vi "Autonomous Independent.vi"() -> ()   [LabVIEW 2011]
doc: "This VI is called when autonomous begins, and will automatically be terminated when autonomous ends. You can carry out timed or sensor driven robot movement independently without needing to return to the caller."
uses:
  <vilib>/Rock Robotics/WPI/Relay/WPI_RelayValue.ctl
  Robot Global Data.vi
panel:
  in  "Recording Auton":bool
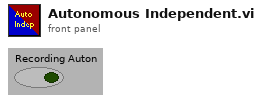
[diagram p1: front panel]
types:
  T1 = typedef "WPI_MotorControlDeviceRef.ctl" = cluster{"DeviceStatus":errorcluster, "Type":enum16{"PWM", "CAN"}, "PWM":cluster{"Digital Module":T2, "PWM Channel":T3, "DeadBand":T4}, "CAN":cluster{"Device Number":u8, "Control Mode":T5, "Semaphore":T6, "Max Vout":dbl}, "Invert":bool, "TransformRef":T7, "InvTransformRef":T7}
  T2 = typedef "FPGA_TypedefDigitalModule.ctl" = enum16{"Digital Module 1", "Digital Module 2"}
  T3 = typedef "FPGA_DIOPWMChannel.ctl" = enum8{"PWM 1", "PWM 2", "PWM 3", "PWM 4", "PWM 5", "PWM 6", "PWM 7", "PWM 8", "PWM 9", "PWM 10", "Invalid"}
  T4 = typedef "WPI_PWMDeadband.ctl" = cluster{"Name":string, "maxPositivePwm":i32, "minPositivePwm":i32, "centerPwm":i32, "maxNegativePwm":i32, "minNegativePwm":i32, "angularRange":u16}
  T5 = typedef "WPI_CANJaguar_ControlMode.ctl" = enum8{"Percent VBus", "Current", "Speed", "Position", "Voltage"}
  T6 = typedef "Semaphore RefNum" = refnum<k1>
  T7 = typedef "WPI_PWMTransform_ConPane.ctl" = refnum<vi>
  T8 = typedef "WPI_ServoDeviceRef.ctl" = cluster{"DeviceStatus":errorcluster, "Digital Module":T2, "PWM Channel":T3, "DeadBand":T4}
  T9 = typedef "WPI_RelayValue.ctl" = enum16{"Off", "On", "Forward", "Reverse"}
  T10 = typedef "WPI_RelayDevRef.ctl" = cluster{"DevStatus":errorcluster, "Relay Channel":T11, "Digital Module":T2, "Relay Direction":T12}
  T11 = typedef "FPGA_DIORelayChannel.ctl" = enum8{"Relay 1", "Relay 2", "Relay 3", "Relay 4", "Relay 5", "Relay 6", "Relay 7", "Relay 8", "Invalid"}
  T12 = typedef "WPI_RelayDirection.ctl" = enum16{"Both directions", "Forward only", "Reverse only"}
  T13 = typedef "WPI_DigitalInputDevRef.ctl" = cluster{"DevStatus":errorcluster, "DIO Channel":T14, "Digital Module":T2}
  T14 = typedef "FPGA_DIOChannel.ctl" = enum8{"DIO 1", "DIO 2", "DIO 3", "DIO 4", "DIO 5", "DIO 6", "DIO 7", "DIO 8", "DIO 9", "DIO 10", "DIO 11", "DIO 12", "DIO 13", "DIO 14", "Invalid"}
  T15 = typedef "WPI_EncoderDevRef.ctl" = cluster{"DevStatus":errorcluster, "EncoderIndex":T16, "CounterIndex":T17, "DistancePerCount":dbl, "Decoding Type":T18}
  T16 = typedef "FPGA_EncoderIdx.ctl" = enum8{"Enc 0", "Enc 1", "Enc 2", "Enc 3", "Invalid"}
  T17 = typedef "FPGA_CounterCtrSystemIndex.ctl" = enum8{"Ctr 0", "Ctr 1", "Ctr 2", "Ctr 3", "Ctr 4", "Ctr 5", "Ctr 6", "Ctr 7", "Invalid"}
  T18 = typedef "WPI_EncoderType.ctl" = enum16{"1x", "2x", "4x"}
  T19 = typedef "WPI_GyroDevRef.ctl" = cluster{"DevStatus":errorcluster, "Analog Module":T20, "Analog Channel":T21, "Offset":dbl, "Gain (VoltsPerDegree/Second)":dbl}
  T20 = typedef "FPGA_TypedefAnalogModule.ctl" = enum16{"Analog Module 1", "Analog Module 2"}
  T21 = typedef "FPGA_AIChannel.ctl" = enum8{"AI 1", "AI 2", "AI 3", "AI 4", "AI 5", "AI 6", "AI 7", "AI 8", "Invalid"}
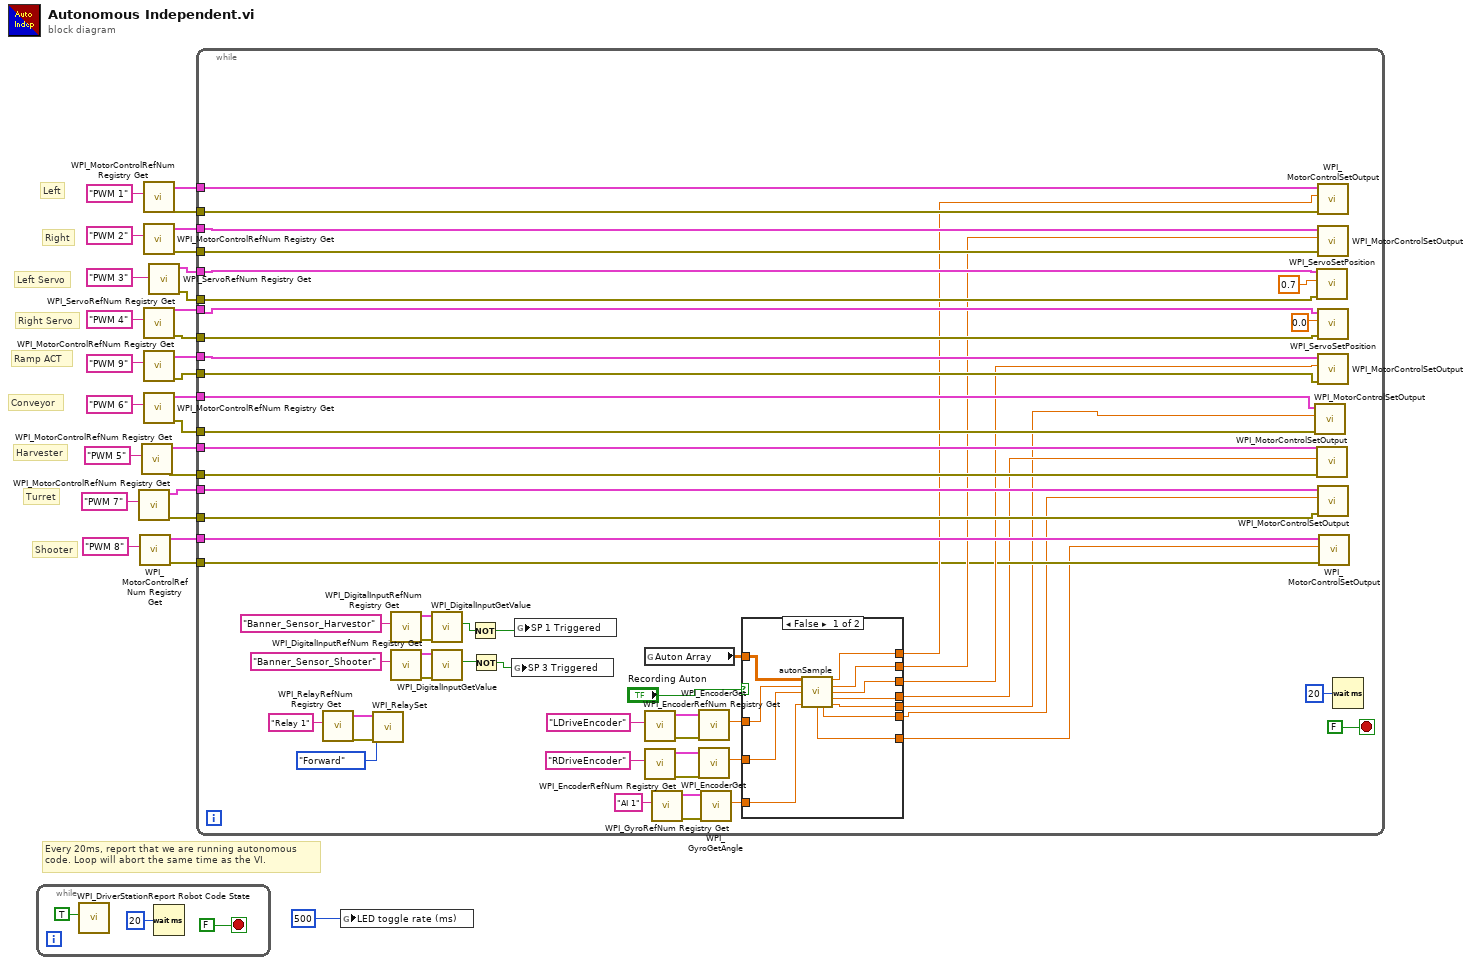
[diagram p0: block diagram]
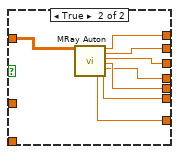
[diagram p2: hidden frame]
diagram:
  # "Shooter"
  # "Turret"
  # "Conveyor"
  # "Harvester"
  # "Ramp ACT"
  # "Right Servo"
  # "Left Servo"
  # "Right"
  # "Left"
  # "Every 20ms, report that we are running autonomous\ncode. Loop will abort the same time as the VI."
  n1 = while {
    stop <- FALSE stop-if-true
    n2 = call <vilib>:"WPI_DriverStationReport Robot Code State.vi"("Autonomous"=TRUE) -> ()  [unwired: 10 in, 1 out]
    n3 = Wait (ms)(milliseconds to wait=u32 20) -> ()  [unwired: 1 out]
  }
  n4 = call <vilib>:"WPI_MotorControlRefNum Registry Get.vi"("refnum name"="PWM 7") -> ("error out"=w8:errorcluster, "MotorControlDevRef"=w9:T1)  [unwired: 9 in]
  n5 = call <vilib>:"WPI_MotorControlRefNum Registry Get.vi"("refnum name"="PWM 8") -> ("error out"=w6:errorcluster, "MotorControlDevRef"=w7:T1)  [unwired: 9 in]
  n6 = call <vilib>:"WPI_MotorControlRefNum Registry Get.vi"("refnum name"="PWM 5") -> ("error out"=w10:errorcluster, "MotorControlDevRef"=w11:T1)  [unwired: 9 in]
  n7 = call <vilib>:"WPI_MotorControlRefNum Registry Get.vi"("refnum name"="PWM 1") -> ("error out"=w1:errorcluster, "MotorControlDevRef"=w23:T1)  [unwired: 9 in]
  n8 = call <vilib>:"WPI_MotorControlRefNum Registry Get.vi"("refnum name"="PWM 2") -> ("error out"=w2:errorcluster, "MotorControlDevRef"=w22:T1)  [unwired: 9 in]
  n9 = call <vilib>:"WPI_ServoRefNum Registry Get.vi"("refnum name"="PWM 4") -> ("error out"=w4:errorcluster, "ServoDeviceRef"=w21:T8)  [unwired: 9 in]
  n10 = call <vilib>:"WPI_MotorControlRefNum Registry Get.vi"("refnum name"="PWM 9") -> ("error out"=w5:errorcluster, "MotorControlDevRef"=w20:T1)  [unwired: 9 in]
  n11 = call <vilib>:"WPI_MotorControlRefNum Registry Get.vi"("refnum name"="PWM 6") -> ("error out"=w15:errorcluster, "MotorControlDevRef"=w16:T1)  [unwired: 9 in]
  n12 = call <vilib>:"WPI_ServoRefNum Registry Get.vi"("refnum name"="PWM 3") -> ("error out"=w3:errorcluster, "ServoDeviceRef"=w18:T8)  [unwired: 9 in]
  n13 = while {
    tunnel: w23 -> [w86]
    tunnel: w22 -> [w85]
    tunnel: w18 -> [w80]
    tunnel: w21 -> [w81]
    tunnel: w20 -> [w84]
    tunnel: w16 -> [w79]
    tunnel: w15 -> [w78]
    tunnel: w11 -> [w77]
    tunnel: w10 -> [w76]
    tunnel: w9 -> [w75]
    tunnel: w8 -> [w74]
    tunnel: w7 -> [w73]
    tunnel: w6 -> [w50]
    tunnel: w5 -> [w72]
    tunnel: w4 -> [w71]
    tunnel: w3 -> [w70]
    tunnel: w2 -> [w69]
    tunnel: w1 -> [w68]
    stop <- FALSE stop-if-true
    n14 = call <vilib>:"WPI_RelayRefNum Registry Get.vi"("refnum name"="Relay 1") -> ("error out"=w38:errorcluster, "RelayDevRef"=w39:T10)  [unwired: 9 in]
    n15 = call <vilib>:"WPI_RelaySet.vi"("error in (no error)"=w38, "RelayValue"=WPI_RelayValue."Forward", "RelayDevRef"=w39) -> ()  [unwired: 7 in, 2 out]
    n16 = call <vilib>:"WPI_DigitalInputRefNum Registry Get.vi"("refnum name"="Banner_Sensor_Harvestor") -> ("error out"=w48:errorcluster, "DigitalInputDevRef"=w49:T13)  [unwired: 9 in]
    n17 = call <vilib>:"WPI_DigitalInputRefNum Registry Get.vi"("refnum name"="Banner_Sensor_Shooter") -> ("error out"=w45:errorcluster, "DigitalInputDevRef"=w44:T13)  [unwired: 9 in]
    n18 = call <vilib>:"WPI_DigitalInputGetValue.vi"("error in (no error)"=w48, "DigitalInputDevRef"=w49) -> ("Value"=w43:bool)  [unwired: 7 in, 2 out]
    n19 = call <vilib>:"WPI_DigitalInputGetValue.vi"("error in (no error)"=w45, "DigitalInputDevRef"=w44) -> ("Value"=w41:bool)  [unwired: 7 in, 2 out]
    n20 = Not(x=w43) -> (.not. x?=w42:bool)
    n21 = Not(x=w41) -> (.not. x?=w40:bool)
    n22 = global write "Robot Global Data.vi" "SP 3 Triggered"(w40) -> ()
    n23 = global write "Robot Global Data.vi" "SP 1 Triggered"(w42) -> ()
    n24 = global read "Robot Global Data.vi" "Auton Array"() -> (w67:dbl[][])
    n25 = call <vilib>:"WPI_EncoderRefNum Registry Get.vi"("refnum name"="LDriveEncoder") -> ("error out"=w61:errorcluster, "EncoderDevRef"=w62:T15)  [unwired: 9 in]
    n26 = call <vilib>:"WPI_EncoderRefNum Registry Get.vi"("refnum name"="RDriveEncoder") -> ("error out"=w51:errorcluster, "EncoderDevRef"=w53:T15)  [unwired: 9 in]
    n27 = call <vilib>:"WPI_GyroRefNum Registry Get.vi"("refnum name"="AI 1") -> ("error out"=w59:errorcluster, "GyroDevRef"=w60:T19)  [unwired: 9 in]
    n28 = call <vilib>:"WPI_EncoderGet.vi"("error in (no error)"=w61, "EncoderDevRef"=w62) -> ("Distance"=w55:dbl)  [unwired: 4 in, 5 out]
    n29 = call <vilib>:"WPI_EncoderGet.vi"("error in (no error)"=w51, "EncoderDevRef"=w53) -> ("Distance"=w54:dbl)  [unwired: 4 in, 5 out]
    n30 = call <vilib>:"WPI_GyroGetAngle.vi"("error in (no error)"=w59, "GyroDevRef"=w60) -> ("Angle"=w56:dbl)  [unwired: 6 in, 3 out]
    n31 = case shown="False" "Recording Auton" {
      tunnel: w67 -> [w99 w107]
      tunnel: [w95 w106] -> w66
      tunnel: [w94 w105] -> w65
      tunnel: [w93 w104] -> w64
      tunnel: w56 -> [w97 _]
      tunnel: w55 -> [w98 _]
      tunnel: w54 -> [w96 _]
      tunnel: [w92 w102] -> w35
      tunnel: [w91 w103] -> w34
      tunnel: [w90 w101] -> w33
      tunnel: [w89 w100] -> w32
      frame False {
        n32 = call "autonSample.vi"("Auton Array"=w99, "LeftEncoder"=w98, "RightEncoder"=w96, "MeasuredHeading"=w97) -> ("Left Drive"=w95:dbl, "Right Drive"=w94:dbl, "Ramp ACT motor"=w93:dbl, "Harvester"=w92:dbl, "Shooter motor output"=w89:dbl, "Turret Rotation"=w90:dbl, "Convyeor"=w91:dbl)  [unwired: 5 in]
      }
      frame True {
        n33 = call "MRay Auton.vi"("Auton Array"=w107) -> ("Shooter"=w100:dbl, "Left Drive"=w106:dbl, "Right Drive"=w105:dbl, "Ramp ACT motor"=w104:dbl, "Conveyor"=w103:dbl, "Harvester"=w102:dbl, "Turret Rotation"=w101:dbl)  [unwired: 12 in]
      }
    }
    n34 = call <vilib>:"WPI_MotorControlSetOutput.vi"("error in (no error)"=w78, "Output"=w34, "MotorControlDevRef"=w79) -> ()  [unwired: 7 in, 2 out]
    n35 = call <vilib>:"WPI_ServoSetPosition.vi"("error in (no error)"=w70, "Position"=0.7 ("Output"), "ServoDeviceRef"=w80) -> ()  [unwired: 7 in, 2 out]
    n36 = call <vilib>:"WPI_MotorControlSetOutput.vi"("error in (no error)"=w76, "Output"=w35, "MotorControlDevRef"=w77) -> ()  [unwired: 7 in, 2 out]
    n37 = call <vilib>:"WPI_MotorControlSetOutput.vi"("error in (no error)"=w68, "Output"=w66, "MotorControlDevRef"=w86) -> ()  [unwired: 7 in, 2 out]
    n38 = call <vilib>:"WPI_MotorControlSetOutput.vi"("error in (no error)"=w69, "Output"=w65, "MotorControlDevRef"=w85) -> ()  [unwired: 7 in, 2 out]
    n39 = call <vilib>:"WPI_ServoSetPosition.vi"("error in (no error)"=w71, "Position"=0.0 ("Output"), "ServoDeviceRef"=w81) -> ()  [unwired: 7 in, 2 out]
    n40 = call <vilib>:"WPI_MotorControlSetOutput.vi"("error in (no error)"=w72, "Output"=w64, "MotorControlDevRef"=w84) -> ()  [unwired: 7 in, 2 out]
    n41 = call <vilib>:"WPI_MotorControlSetOutput.vi"("error in (no error)"=w74, "Output"=w33, "MotorControlDevRef"=w75) -> ()  [unwired: 7 in, 2 out]
    n42 = call <vilib>:"WPI_MotorControlSetOutput.vi"("error in (no error)"=w50, "Output"=w32, "MotorControlDevRef"=w73) -> ()  [unwired: 7 in, 2 out]
    n43 = Wait (ms)(milliseconds to wait=u32 20) -> ()  [unwired: 1 out]
  }
  n44 = global write "Robot Global Data.vi" "LED toggle rate (ms)"(u32 500 ("LED ms toggle rate")) -> ()
